vi "ResetAndDefineConstants.vi"   [LabVIEW 2020]
doc: "This VI sets constants and resets the global variables."
uses:
  robotconstants.vi
  robotoutputs.vi
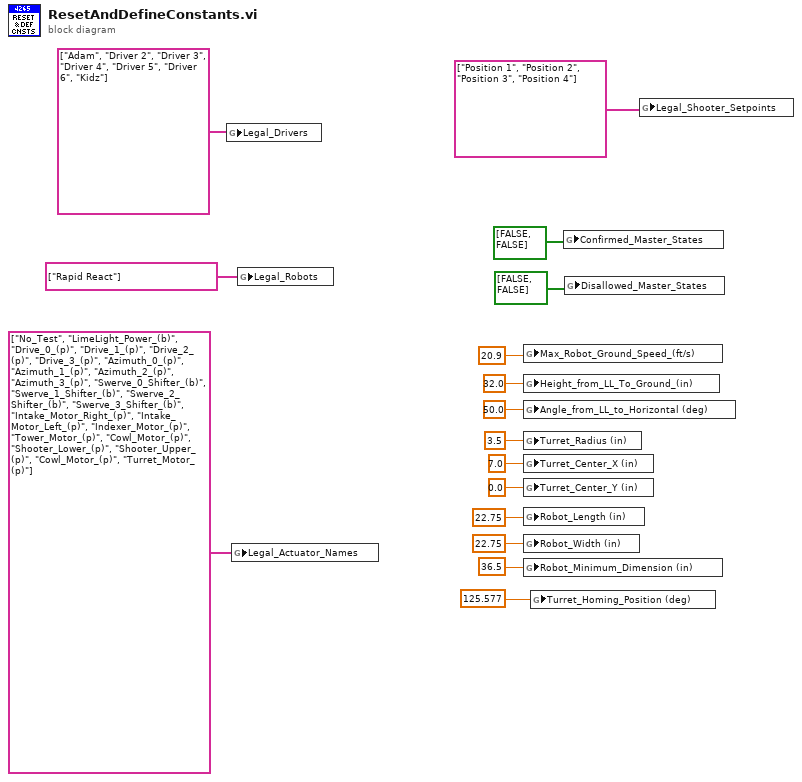
[diagram p0: block diagram]
diagram:
  n1 = global write "robotconstants.vi" "Legal_Drivers"(string[] ["Adam", "Driver 2", "Driver 3", "Driver 4", "Driver 5", "Driver 6", "Kidz"] ("appended array")) -> ()
  n2 = global write "robotconstants.vi" "Legal_Actuator_Names"(string[] ["No_Test", "LimeLight_Power_(b)", "Drive_0_(p)", "Drive_1_(p)", "Drive_2_(p)", "Drive_3_(p)", "Azimuth_0_(p)", "Azimuth_1_(p)", "Azimuth_2_(p)", "Azimuth_3_(p)", "Swerve_0_Shifter_(b)", "Swerve_1_Shifter_(b)", "Swerve_2_Shifter_(b)", "Swerve_3_Shifter_(b)", "Intake_Motor_Right_(p)", "Intake_Motor_Left_(p)", "Indexer_Motor_(p)", "Tower_Motor_(p)", "Cowl_Motor_(p)", "Shooter_Lower_(p)", "Shooter_Upper_(p)", "Cowl_Motor_(p)", "Turret_Motor_(p)"] ("appended array")) -> ()
  n3 = global write "robotconstants.vi" "Legal_Robots"(string[] ["Rapid React"] ("Legal_Actuator_Names")) -> ()
  n4 = global write "robotconstants.vi" "Max_Robot_Ground_Speed_(ft/s)"(20.9 ("Max_Robot_Ground_Speed_(ft/s)")) -> ()
  n5 = global write "robotconstants.vi" "Height_from_LL_To_Ground_(in)"(32.0 ("Max_Robot_Ground_Speed_(ft/s)")) -> ()
  n6 = global write "robotconstants.vi" "Angle_from_LL_to_Horizontal (deg)"(50.0 ("Max_Robot_Ground_Speed_(ft/s)")) -> ()
  n7 = global write "robotconstants.vi" "Turret_Radius (in)"(3.5 ("Max_Robot_Ground_Speed_(ft/s)")) -> ()
  n8 = global write "robotconstants.vi" "Turret_Center_X (in)"(7.0 ("Max_Robot_Ground_Speed_(ft/s)")) -> ()
  n9 = global write "robotconstants.vi" "Turret_Center_Y (in)"(0.0 ("Max_Robot_Ground_Speed_(ft/s)")) -> ()
  n10 = global write "robotconstants.vi" "Robot_Length (in)"(22.75 ("Robot_Length (in)")) -> ()
  n11 = global write "robotconstants.vi" "Robot_Width (in)"(22.75 ("Robot_Length (in)")) -> ()
  n12 = global write "robotconstants.vi" "Robot_Minimum_Dimension (in)"(36.5 ("Robot_Length (in)")) -> ()
  n13 = global write "robotconstants.vi" "Turret_Homing_Position (deg)"(125.577 ("Robot_Length (in)")) -> ()
  n14 = global write "robotoutputs.vi" "Confirmed_Master_States"(bool[] [FALSE, FALSE] ("Disallowed_Master_States")) -> ()
  n15 = global write "robotoutputs.vi" "Disallowed_Master_States"(bool[] [FALSE, FALSE] ("Disallowed_Master_States")) -> ()
  n16 = global write "robotconstants.vi" "Legal_Shooter_Setpoints"(string[] ["Position 1", "Position 2", "Position 3", "Position 4"] ("appended array")) -> ()
